vi "TemplateGUI_MainGUIActive.vi"(8 "Error In":errorcluster, 11 "reference in":refnum<class "TemplateGUI.lvclass">) -> (0 "Error Out":errorcluster, 3 "reference in":refnum<class "TemplateGUI.lvclass">)   [LabVIEW 2021, in "TemplateGUI.lvlib" / "TemplateGUI.lvclass"]
uses:
  TemplateGUI.lvclass
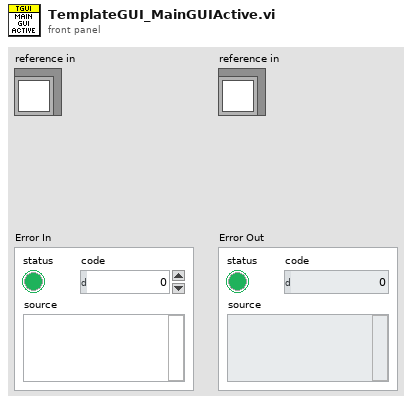
[diagram p1: front panel]
types:
  T1 = typedef "TemplateGUI.lvlib/TemplateGUI.lvclass/ObjectAttributes.ctl" = cluster{"Interfaces":cluster{"Dummys":refnum<class>}, "Locals":cluster{"MainGUIActive":refnum<queue>}, "Persistent":cluster{"Dummy":bool}}
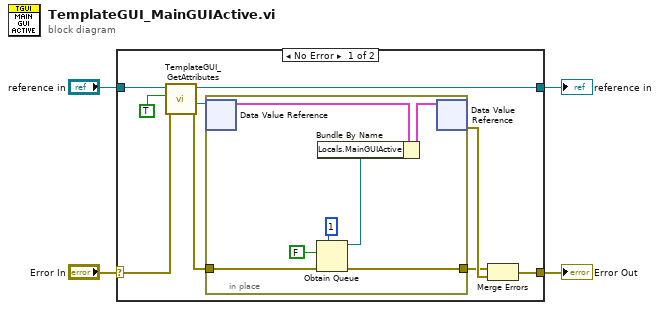
[diagram p0: block diagram]
diagram:
  n1 = case shown="No Error" "Error In" {
    selector: "Error In" -> [w11 w22]
    tunnel: [w7 w22] -> w3
    tunnel: [w12 w21] -> w1
    tunnel: "reference in" -> [w13 w21]
    frame No Error {
      n2 = call "TemplateGUI_GetAttributes.vi"("error in (no error)"=w11, "OnlyGetDvrReference(False)"=TRUE, "reference in"=w13) -> ("error out"=w6:errorcluster, "DataRef"=w8:refnum<data-value>, "reference out"=w12:refnum<class "TemplateGUI.lvclass">)  [unwired: 5 in, 1 out]
      n3 = in-place {
        in-place-border: w6 -> [w16]
        in-place-border: [w15] -> w5
        n4 = in-place-dvr #1(w8) -> (w19:T1)  [unwired: 1 out]
        n5 = Obtain Queue(max queue size (-1, unlimited)=1, element data type=FALSE, error in (no error)=w16) -> (queue out=w14:refnum<queue>, error out=w15:errorcluster)  [unwired: 2 in, 1 out]
        n6 = Bundle By Name(cluster=w19, "Locals.MainGUIActive"=w14) -> (w20:T1)
        n7 = in-place-dvr #1(w20) -> (w9:errorcluster)  [unwired: 1 out]
      }
      n8 = Merge Errors(w5, w9) -> (w7:errorcluster)
    }
    frame Error {
    }
  }
  "Error Out" <- w3
  "reference in" <- w1
